vi "Untitled 1.vi"() -> ()   [LabVIEW 2015]
panel:
  out "data":dbl[][](array[numeric])
  in  "stop":bool
  out "Waveform Chart":dbl(graph)
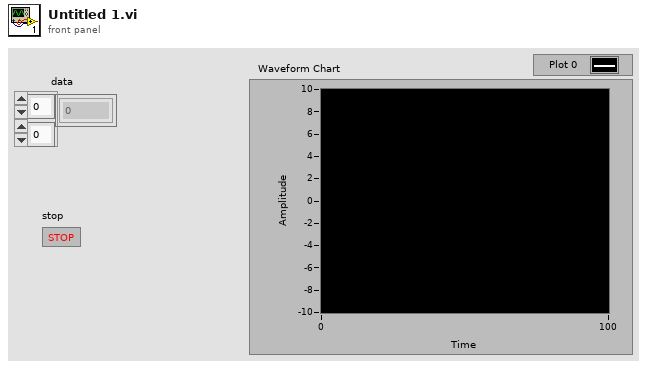
[diagram p1: front panel]
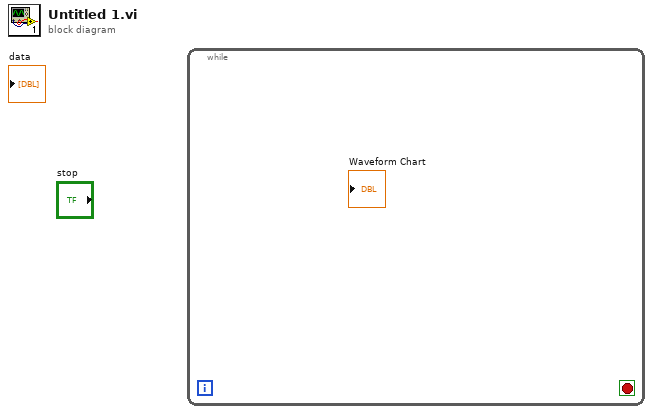
[diagram p0: block diagram]
diagram:
  n1 = while {
    stop <- _ stop-if-true
  }
